vi "log_error.vi"(8 "error in":errorcluster, 10 "Elog Properties":T5={"Logbook"="CTS", "Author"="Hampai", "Type"="Experiment", "Category"="General", "Severity"="Log"}, 11 "VI Refnum":refnum<vi>) -> (0 "error out":errorcluster)   [LabVIEW 2023]
uses:
  support.project/elog/control/logbook.ctl
  support.project/elog/control/type.ctl
  support.project/elog/control/category.ctl
  support.project/elog/control/severity.ctl
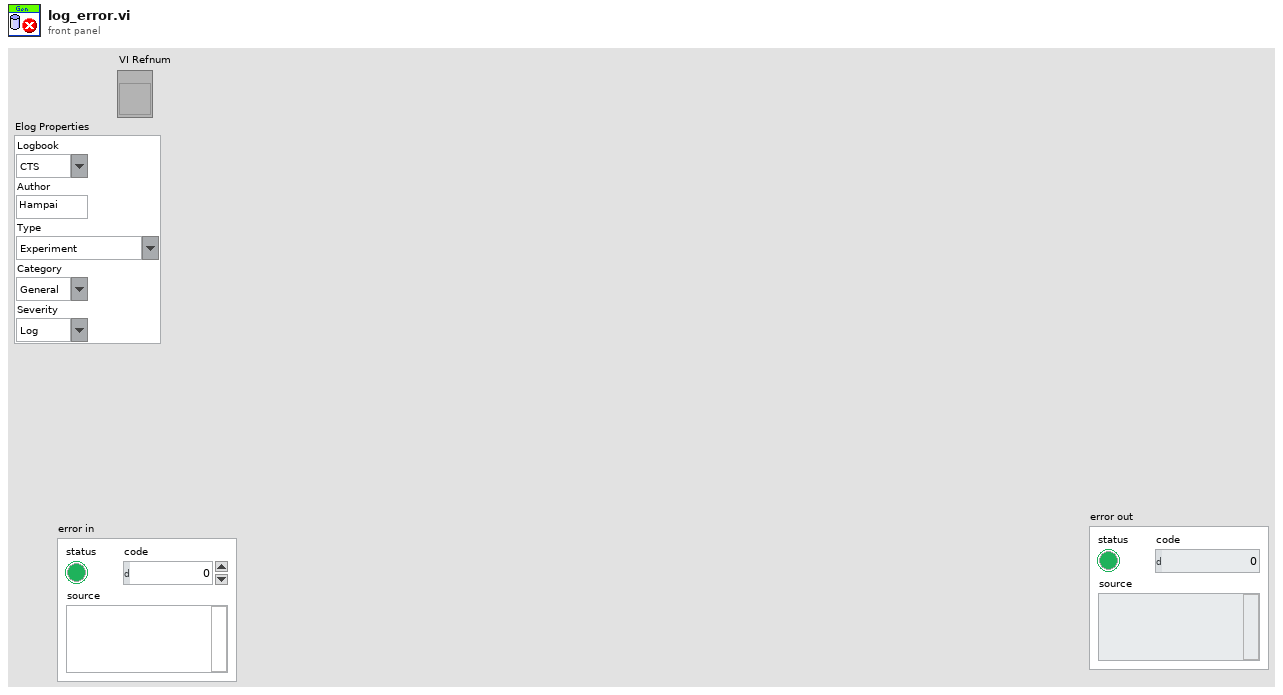
[diagram p1: front panel]
types:
  T1 = typedef "logbook.ctl" = string
  T2 = typedef "type.ctl" = string
  T3 = typedef "category.ctl" = string
  T4 = typedef "severity.ctl" = string
  T5 = cluster{"Logbook":T1, "Author":string, "Type":T2, "Category":T3, "Severity":T4}
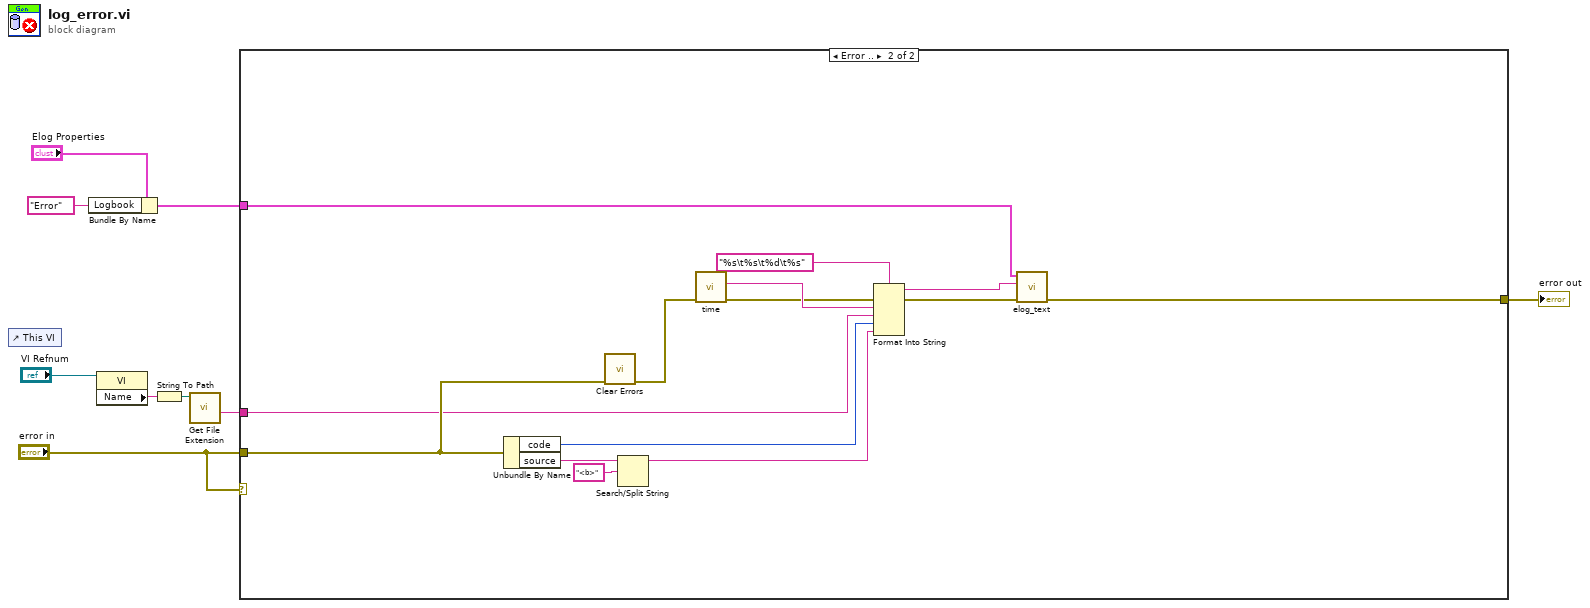
[diagram p0: block diagram]
diagram:
  n1 = control-ref of="This VI"() -> ()  [unwired: 1 out]
  n2 = Bundle By Name(cluster="Elog Properties", "Logbook"=T1 "Error") -> (w1:T5)
  n3 = property class="VI"(reference="VI Refnum") -> ("Name"=w7:string)  [unwired: 1 in, 2 out]
  n4 = String To Path(string=w7) -> (path=w8:path)
  n5 = call <vilib>:"Get File Extension.vi"("file"=w8) -> ("filename without extension"=w6:string)  [unwired: 1 in, 9 out]
  n6 = case shown="Error .." "error in" {
    tunnel: "error in" -> [w10 w22]
    tunnel: [w10 w13] -> w9
    tunnel: w6 -> [_ w19]
    tunnel: w1 -> [_ w11]
    frame No Error {
    }
    frame Error {
      n7 = Unbundle By Name(w22) -> ("code"=w21:i32, "source"=w23:string)
      n8 = call <vilib>:"Clear Errors.vi"("error in (no error)"=w22) -> ("error out"=w16:errorcluster)  [unwired: 5 in, 1 out]
      n9 = Search/Split String(string=w23, search string/char (-)="<b>") -> (substring before match=w20:string)  [unwired: 1 in, 2 out]
      n10 = call "time.vi"("Error In"=w16) -> ("Error Out"=w15:errorcluster, "datetime"=w17:string)  [unwired: 6 in, 3 out]
      n11 = Format Into String(format string="%s\t%s\t%d\t%s", error in=w15, w17, w19, w21, w20) -> (resulting string=w12:string, error out=w14:errorcluster)  [unwired: 1 in]
      n12 = call "elog_text.vi"("error in (no error)"=w14, "Text to log"=w12, "Elog Properties"=w11) -> ("error out"=w13:errorcluster)  [unwired: 8 in]
    }
  }
  "error out" <- w9
